vi "Edit Project File Build Spec Destinations.vi"(7 "xml name":string, 8 "error in":errorcluster, 9 "CD lvproj name":string, 10 "CD name":string, 11 "custom device path":path) -> (0 "error out":errorcluster, 3 "custom device path out":path)   [LabVIEW 2020, in "Template Tool.lvlib"]
uses:
  Template Tool.lvlib
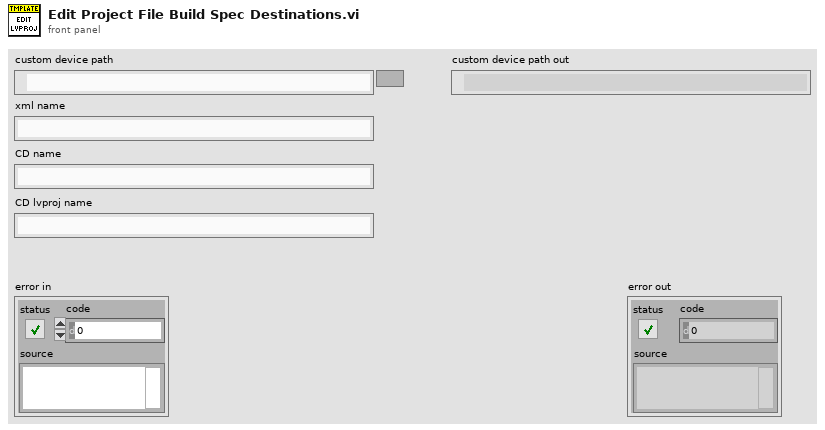
[diagram p1: front panel]
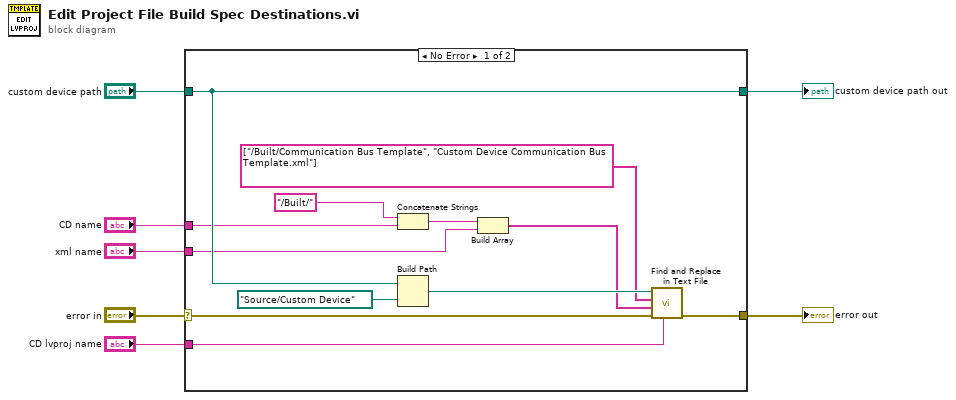
[diagram p0: block diagram]
diagram:
  n1 = case shown="No Error" "error in" {
    selector: "error in" -> [w17 w20]
    tunnel: "custom device path" -> [w16 w21]
    tunnel: [w15 w20] -> w7
    tunnel: [w16 w21] -> w4
    tunnel: "CD name" -> [w10 _]
    tunnel: "xml name" -> [w9 _]
    tunnel: "CD lvproj name" -> [w8 _]
    frame No Error {
      n2 = Concatenate Strings("/Built/" ("string"), w10) -> (w13:string)
      n3 = Build Path(base path=w16, name or relative path=path "Source/Custom Device") -> (appended path=w14:path)
      n4 = Build Array(w13, w9) -> (w11:string[])
      n5 = call "Find and Replace in Text File.vi"("file name"=w8, "error in"=w17, "replace array"=w11, "find array"=string[] ["/Built/Communication Bus Template", "Custom Device Communication Bus Template.xml"], "folder path"=w14) -> ("error out"=w15:errorcluster)  [unwired: 5 in, 1 out]
    }
    frame Error {
    }
  }
  "error out" <- w7
  "custom device path out" <- w4
